vi "Read Init.vi"(8 "error in (no error)":errorcluster, 11 "NMR in":refnum<class "NMR.lvclass">) -> (0 "error out":errorcluster, 2 "Init":bool, 3 "NMR out":refnum<class "NMR.lvclass">)   [LabVIEW 2011, in "NMR.lvclass"]
uses:
  NMR.lvclass
  NMR.lvclass/NMR.ctl
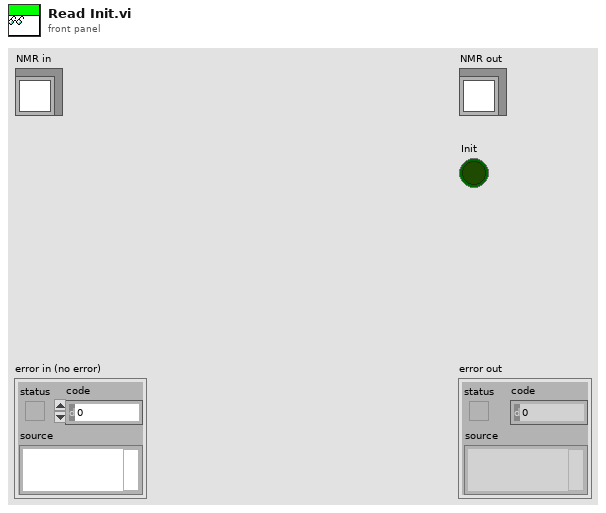
[diagram p1: front panel]
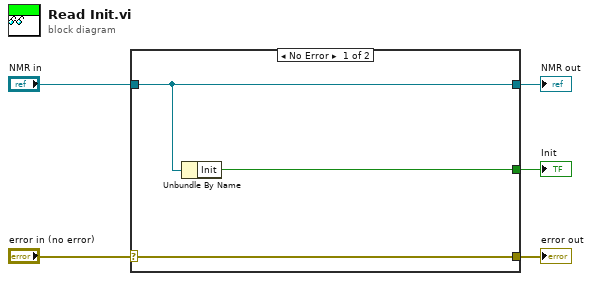
[diagram p0: block diagram]
diagram:
  n1 = case shown="No Error" "error in (no error)" {
    selector: "error in (no error)" -> [w8 w9]
    tunnel: [w8 w9] -> w4
    tunnel: [w7 w10] -> w2
    tunnel: "NMR in" -> [w7 w10]
    tunnel: [w6 _] -> w1
    frame No Error {
      n2 = Unbundle By Name(w7) -> ("Init"=w6:bool)
    }
    frame Error {
    }
  }
  "error out" <- w4
  "NMR out" <- w2
  "Init" <- w1
